vi "create_stim_task.vi"(8 "error in":errorcluster, 11 "Stim protocol":T1={"Frequency"=0.01, "Pulse duration"=0.001, "Stop after"=0.0} {"Stop after" min=0.0 max=500.0; "Pulse duration" min=0.001 max=0.1; "Frequency" min=0.01 max=200.0 step=1.0}) -> (0 "error out":errorcluster, 3 "task out":refnum<k21>)   [LabVIEW 2010]
uses:
  typedefs/stim_protocol_cluster.ctl
  <vilib>/DAQmx/create/channels.llb/DAQmx Create Channel (AO-Voltage-Basic).vi
  <vilib>/DAQmx/configure/timing.llb/DAQmx Timing (Sample Clock).vi
  Program Files/National Instruments/LabVIEW 2010/resource/objmgr/daqmx.rc
panel:
  # "0 for manual stop"
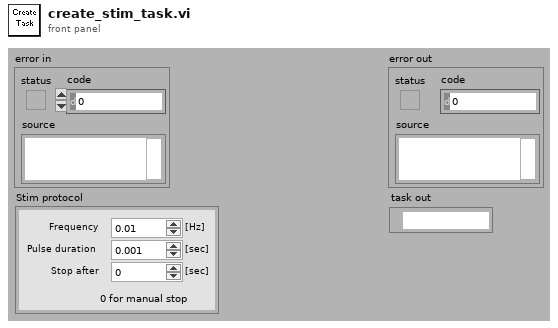
[diagram p1: front panel]
types:
  T1 = typedef "stim_protocol_cluster.ctl" = cluster{"Frequency":dbl, "Pulse duration":dbl, "Stop after":dbl}
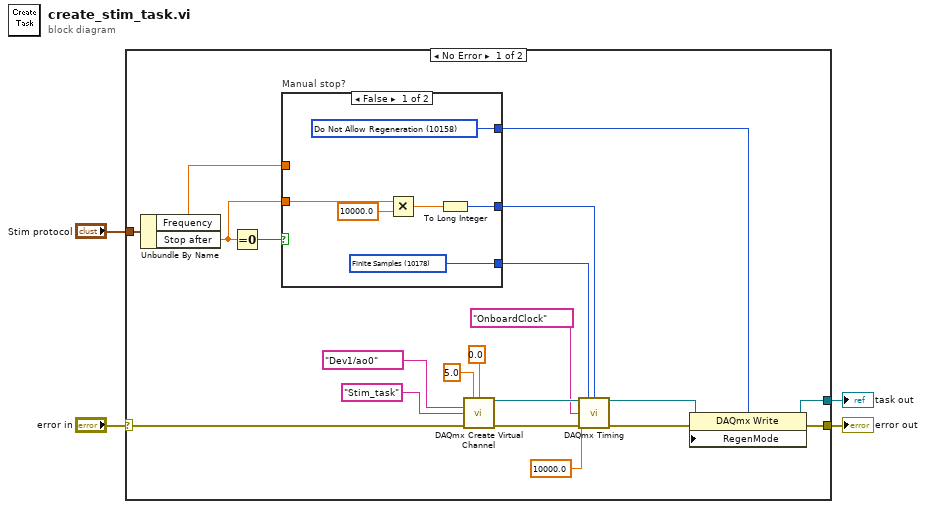
[diagram p0: block diagram]
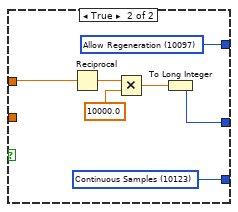
[diagram p2: hidden frame]
diagram:
  n1 = case shown="No Error" "error in" {
    selector: "error in" -> [w5 w38]
    tunnel: "Stim protocol" -> [w17 _]
    tunnel: [w8 w38] -> w3
    tunnel: [w7 _] -> w2
    frame No Error {
      n2 = Unbundle By Name(w17) -> ("Frequency"=w12:dbl, "Stop after"=w15:dbl)
      n3 = Equal To 0?(x=w15) -> (x = 0?=w16:bool)
      n4 = case "Manual stop?" shown="False" w16 {
        tunnel: w15 -> [w30 _]
        tunnel: [w28 w37] -> w14
        tunnel: [w26 w32] -> w13
        tunnel: w12 -> [_ w36]
        tunnel: [w25 w31] -> w9
        frame False {
          w25 = 10158 items=["Allow Regeneration"=10097, "Do Not Allow Regeneration"=10158] ("RegenMode")
          w28 = 10178 items=["Finite Samples"=10178, "Continuous Samples"=10123, "Hardware Timed Single Point"=12522] ("sample mode")
          n5 = Multiply(x=w30, y=10000.0) -> (x*y=w27:dbl)
          n6 = To Long Integer(number=w27) -> (32bit integer=w26:i32)
        }
        frame True {
          w31 = 10097 items=["Allow Regeneration"=10097, "Do Not Allow Regeneration"=10158] ("RegenMode")
          w37 = 10123 items=["Finite Samples"=10178, "Continuous Samples"=10123, "Hardware Timed Single Point"=12522] ("sample mode")
          n7 = Reciprocal(x=w36) -> (1/x=w35:dbl)
          n8 = Multiply(x=w35, y=10000.0) -> (x*y=w33:dbl)
          n9 = To Long Integer(number=w33) -> (32bit integer=w32:i32)
        }
      }
      n10 = call-poly <vilib>:"DAQmx Create Virtual Channel.vi"("maximum value"=5.0, "minimum value"=0.0, "physical channels"=tag "Dev1/ao0", "name to assign"="Stim_task", "error in"=w5) -> ("task out"=w19:refnum<k21>, "error out"=w20:errorcluster)  [unwired: 9 in]
      n11 = call-poly <vilib>:"DAQmx Timing.vi"("task/channels in"=w19, "sample mode"=w14, "samples per channel"=w13, "rate"=10000.0, "source"=tag "OnboardClock", "error in"=w20) -> ("task out"=w10:refnum<k21>, "error out"=w11:errorcluster)  [unwired: 8 in]
      n12 = property class="DAQmx Write"(reference=w10, error in=w11, "RegenMode"=w9) -> (reference out=w7:refnum<k21>, error out=w8:errorcluster)
    }
    frame Error {
    }
  }
  "error out" <- w3
  "task out" <- w2
